vi "Show Windows(輸入密碼).vi"(3 "String 2":string, 8 "error in (no error)":errorcluster) -> (0 "error out":errorcluster, 2 "密碼正確":bool)   [LabVIEW 2015]
uses:
  Read_ini_ArrayStr.vi
panel:
  in  "OK Button":bool
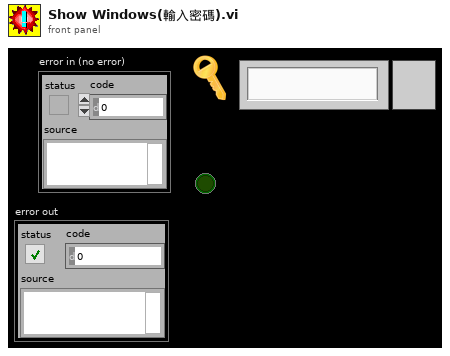
[diagram p1: front panel]
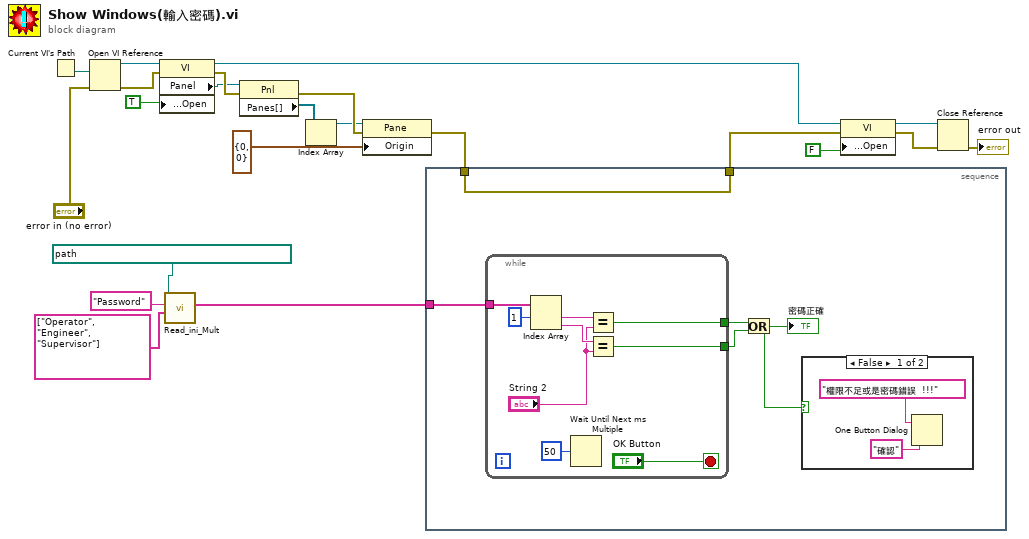
[diagram p0: block diagram]
diagram:
  n1 = Current VI's Path() -> (path=w20:path)
  n2 = Open VI Reference(vi path=w20, error in (no error)="error in (no error)") -> (vi reference=w14:refnum<vi>, error out=w15:errorcluster)  [unwired: 4 in]
  n3 = property class="VI"(reference=w14, error in=w15, "Front Panel.Open"=TRUE ("Front Panel Window:Open")) -> (reference out=w11:refnum<vi>, error out=w21:errorcluster, "Panel"=w19:refnum<vi>)
  n4 = call-poly "Read_ini_Mult.vi"("key names"=string[] ["Operator", "Engineer", "Supervisor"], "section"="Password", "configuration file path"=path "D:/半自動電檢機 Data/Recipe/Default.ini") -> ("ArrayValue"=w1:string[])  [unwired: 7 in, 1 out]
  n5 = property class="Pnl"(reference=w19, error in=w21) -> (error out=w22:errorcluster, "Panes[]"=w16:refnum<vi>[])  [unwired: 1 out]
  n6 = Index Array(array=w16) -> (element=w17:refnum<vi>)  [unwired: 1 in]
  n7 = property class="Pane"(reference=w17, error in=w22, "Origin"=cluster{"Horizontal":i16, "Vertical":i16} {"Horizontal"=0, "Vertical"=0}) -> (error out=w12:errorcluster)  [unwired: 1 out]
  n8 = stacked-sequence {
    tunnel: [w27] -> w8
    tunnel: w12 -> [w27]
    tunnel: w1 -> [w26]
    frame #0 {
      n9 = while {
        tunnel: w26 -> [w36]
        tunnel: [w31] -> w25
        tunnel: [w30] -> w24
        stop <- "OK Button" stop-if-true
        n10 = Index Array(array=w36, index #1=1 ("index")) -> (element #1=w34:string, element #2=w33:string)  [unwired: 1 in]
        n11 = Wait Until Next ms Multiple(millisecond multiple=u32 50) -> ()  [unwired: 1 out]
        n12 = Equal?(x=w34, y="String 2") -> (x = y?=w31:bool)
        n13 = Equal?(x=w33, y="String 2") -> (x = y?=w30:bool)
      }
      n14 = Or(x=w25, y=w24) -> (x .or. y?=w23:bool)
      "密碼正確" <- w23
      n15 = case shown="False" w23 {
        frame False {
          n16 = One Button Dialog(message="權限不足或是密碼錯誤  !!!", button name ("OK")="確認") -> ()  [unwired: 1 out]
        }
        frame True {
        }
      }
    }
  }
  n17 = property class="VI"(reference=w11, error in=w8, "Front Panel.Open"=FALSE ("Front Panel Window:Open")) -> (reference out=w10:refnum<vi>, error out=w7:errorcluster)
  n18 = Close Reference(reference=w10, error in (no error)=w7) -> (error out=→"error out":errorcluster)
